vi "switch screens.vi"(8 "error in (no error)":errorcluster caption="错误输入（无错误）", 11 "DGUS 输入":refnum<class "DGUS.lvclass">) -> (0 "error out":errorcluster caption="错误输出", 2 "字符串":string, 3 "DGUS 输出":refnum<class "DGUS.lvclass">)   [LabVIEW 2016, in "DGUS.lvlib" / "DGUS.lvclass"]
uses:
  DGUS.lvclass
  DGUS.lvclass/DGUS.ctl
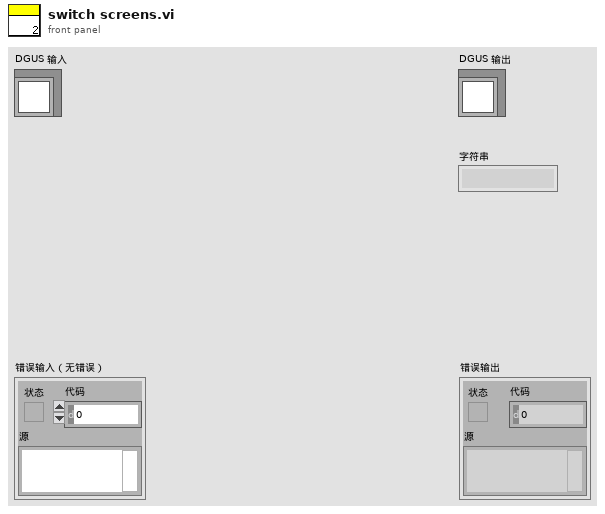
[diagram p1: front panel]
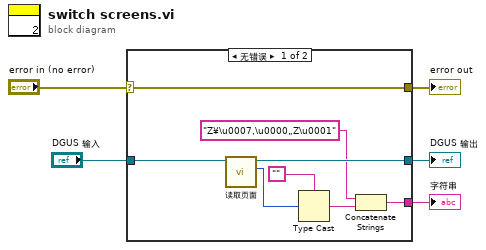
[diagram p0: block diagram]
diagram:
  n1 = case shown="无错误" "error in (no error)" {
    selector: "error in (no error)" -> [w13 w15]
    tunnel: [w13 w15] -> w4
    tunnel: [w11 w14] -> w2
    tunnel: "DGUS 输入" -> [w12 w14]
    tunnel: [w6 _] -> w1
    frame No Error {
      n2 = call "读取页面.vi"("DGUS输入"=w12) -> ("页面"=w10:u16, "DGUS输出"=w11:refnum<class "DGUS.lvclass">)  [unwired: 8 in, 1 out]
      n3 = Type Cast(type="", x=w10) -> (*(type *) &x=w7:string)
      n4 = Concatenate Strings("Z¥\u0007‚\u0000„Z\u0001" ("初始字符串"), w7) -> (w6:string)
    }
    frame Error {
    }
  }
  "error out" <- w4
  "DGUS 输出" <- w2
  "字符串" <- w1
